vi "Meta Data to Variant.vi"(6 "Meta data":string, 8 "Error In":errorcluster, 10 "Section":string, 11 "Value":variant) -> (0 "Error Out":errorcluster, 1 "found?":bool, 2 "deleted path":path, 3 "Variant out":variant)   [LabVIEW 2016]
uses:
  <vilib>/Utility/config.llb/NI_LVConfig.lvlib
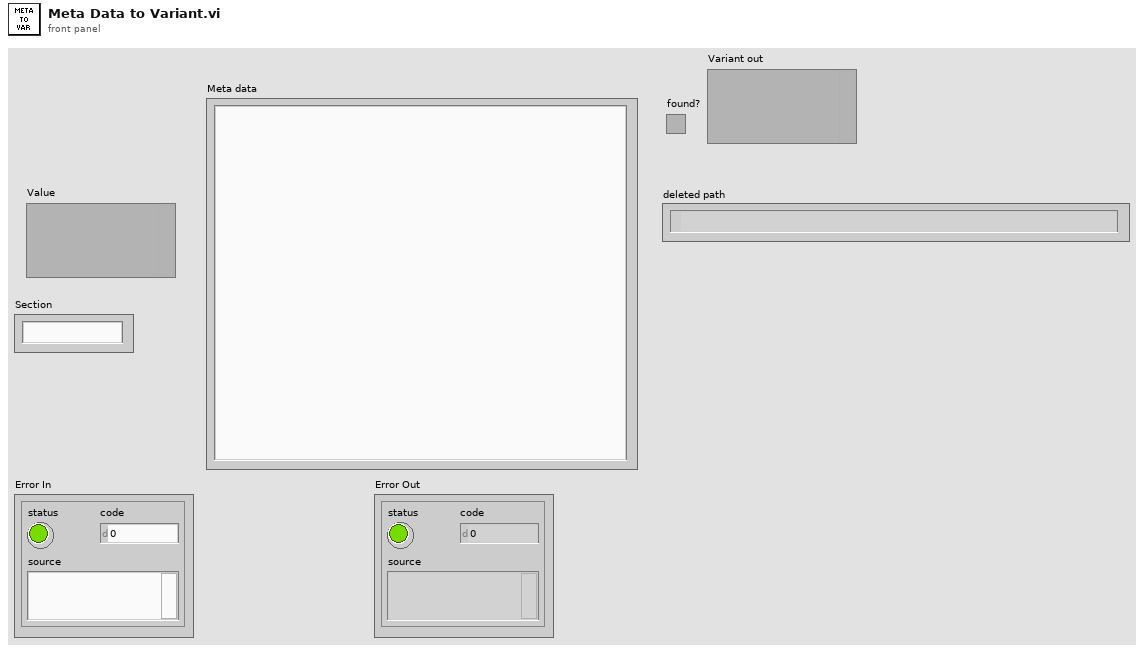
[diagram p1: front panel]
types:
  T1 = typedef "NI_LVConfig.lvlib/Config Data RefNum.ctl" = refnum<k1>
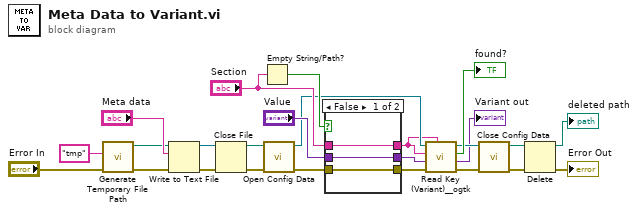
[diagram p0: block diagram]
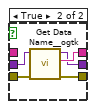
[diagram p2: hidden frame]
diagram:
  n1 = call <vilib>:"Generate Temporary File Path.vi"("error in (no error)"="Error In", "Temporary File Extension (tmp)"="tmp") -> ("error out"=w13:errorcluster, "Unique Temporary File Path"=w14:path)  [unwired: 8 in]
  n2 = Write to Text File(file (use dialog)=w14, text="Meta data", error in=w13) -> (refnum out=w24:refnum<file>, error out=w23:errorcluster)  [unwired: 1 in, 1 out]
  n3 = Close File(refnum=w24, error in=w23) -> (path=w11:path, error out=w12:errorcluster)
  n4 = Empty String/Path?(string/path="Section") -> (empty?=w18:bool)
  n5 = call <vilib>:"Open Config Data.vi"("error in (no error)"=w12, "configuration file path"=w11) -> ("error out"=w17:errorcluster, "refnum"=w9:T1)  [unwired: 7 in, 1 out]
  n6 = case shown="False" w18 {
    tunnel: "Value" -> [w28 w33]
    tunnel: [w26 w32] -> w1
    tunnel: w17 -> [w27 w31]
    tunnel: [w27 w30] -> w8
    tunnel: [w28 w29] -> w10
    tunnel: "Section" -> [w26 _]
    frame False {
    }
    frame True {
      n7 = call <userlib>:"Get Data Name__ogtk.vi"("error in (no error)"=w31, "Data"=w33) -> ("error out"=w30:errorcluster, "Data Name"=w32:string, "Data dup"=w29:variant)  [unwired: 7 in]
    }
  }
  n8 = call <userlib>:"Read Key (Variant)__ogtk.vi"("section"=w1, "error in (no error)"=w8, "type"=w10, "key (optional)"=w1, "refnum"=w9) -> ("error out"=w3:errorcluster, "key-value"=→"Variant out":variant, "found?"=→"found?":bool, "refnum out"=w4:T1)  [unwired: 3 in]
  n9 = call <vilib>:"Close Config Data.vi"("error in (no error)"=w3, "refnum"=w4) -> ("error out"=w6:errorcluster, "file path"=w7:path)  [unwired: 8 in]
  n10 = Delete(path (use dialog)=w7, error in=w6) -> (deleted path=→"deleted path":path, error out=→"Error Out":errorcluster)  [unwired: 3 in, 1 out]
